vi "SP Convert Parameter from String to Cluster.vi"(10 "Parameter String":string) -> (2 "Parameter":T1 {"Stimulus Port" min=1 step=1; "Response Port" min=1 step=1})   [LabVIEW 2011]
uses:
  TypeDefs/SP Parameter.ctl
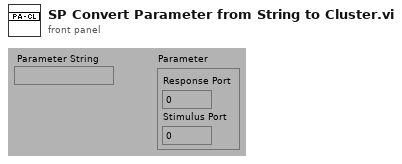
[diagram p1: front panel]
types:
  T1 = typedef "SP Parameter.ctl" = cluster{"Stimulus Port":i8, "Response Port":i8}
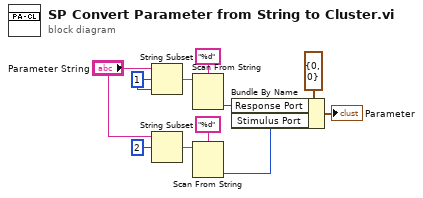
[diagram p0: block diagram]
diagram:
  w7 = 1 ("offset (0)")
  n1 = String Subset(string="Parameter String", offset (0)=w7, length (rest)=w7) -> (substring=w6:string)
  n2 = String Subset(string="Parameter String", offset (0)=2) -> (substring=w4:string)  [unwired: 1 out]
  n3 = Scan From String(format string="%d", input string=w6) -> (output 1=w3:i32)  [unwired: 2 in, 4 out]
  n4 = Scan From String(format string="%d", input string=w4) -> (output 1=w2:i32)  [unwired: 2 in, 4 out]
  n5 = Bundle By Name(cluster=T1 {"Stimulus Port"=0, "Response Port"=0} ("Parameter"), "Response Port"=w3, "Stimulus Port"=w2) -> (→"Parameter":T1)
